vi "Close_COM.vi"(8 "error in (no error)":errorcluster, 11 "USB-87Pn in":refnum<class "USB-87Pn.lvclass">) -> (0 "error out":errorcluster, 3 "USB-87Pn out":refnum<class "USB-87Pn.lvclass">)   [LabVIEW 2019, in "USB-87Pn.lvlib" / "USB-87Pn.lvclass"]
uses:
  USB-87Pn.lvclass
  USB-87Pn.lvclass/USB-87Pn.ctl
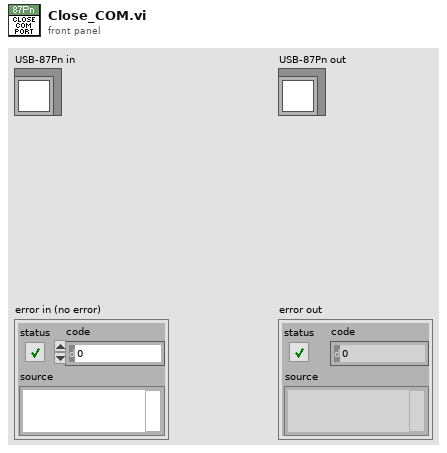
[diagram p1: front panel]
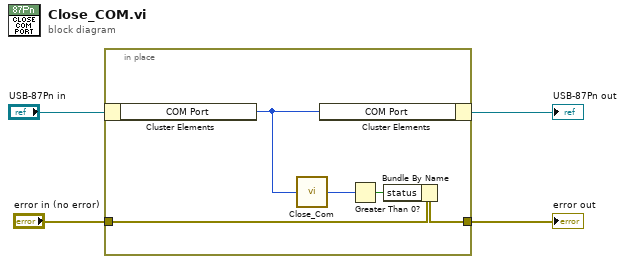
[diagram p0: block diagram]
diagram:
  n1 = in-place {
    in-place-border: "error in (no error)" -> [w8]
    in-place-border: [w7] -> w2
    n2 = in-place-cluster #1("USB-87Pn in") -> ("COM Port"=w6:u8)
    n3 = call "Close_Com.vi"("port number"=w6) -> ("return"=w5:u16)
    n4 = in-place-cluster #1("COM Port"=w6) -> (→"USB-87Pn out":refnum<class "USB-87Pn.lvclass">)
    n5 = Greater Than 0?(x=w5) -> (x > 0?=w9:bool)
    n6 = Bundle By Name(cluster=w8, "status"=w9) -> (w7:errorcluster)
  }
  "error out" <- w2
